vi "Contestant Buzzed.vi"(8 "error in (no error)":errorcluster, 10 "Contestant":i32, 11 "MC Prompt in":refnum<class "MC Prompt.lvclass">) -> (0 "error out":errorcluster, 3 "MC Prompt out":refnum<class "MC Prompt.lvclass">)   [LabVIEW 2021, in "MC Prompt.lvlib" / "MC Prompt.lvclass"]
uses:
  MC Prompt.lvclass
  MC Prompt.lvclass/MC Prompt.ctl
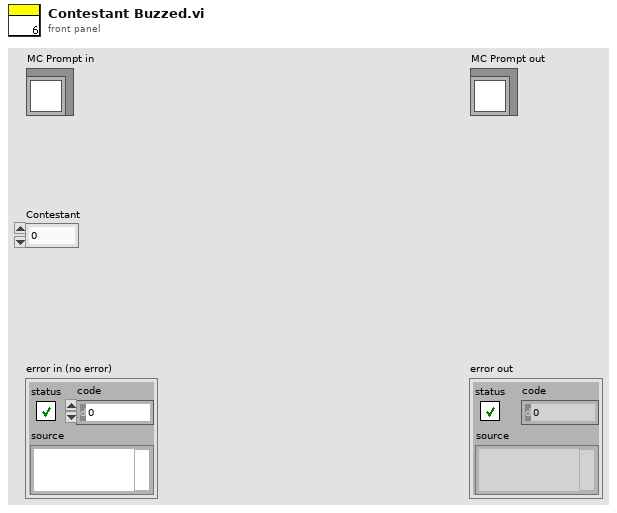
[diagram p1: front panel]
types:
  T1 = enum8{"Enabled", "Disabled", "Disabled and Grayed Out"}
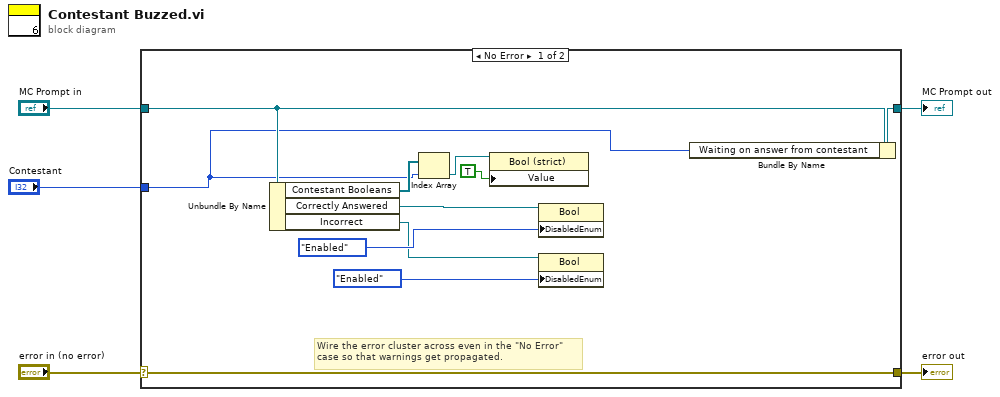
[diagram p0: block diagram]
diagram:
  n1 = case shown="No Error" "error in (no error)" {
    selector: "error in (no error)" -> [w16 w18]
    tunnel: [w16 w18] -> w4
    tunnel: [w7 w17] -> w2
    tunnel: "MC Prompt in" -> [w8 w17]
    tunnel: "Contestant" -> [w6 _]
    frame No Error {
      # "Wire the error cluster across even in the \"No Error\"\ncase so that warnings get propagated."
      n2 = Unbundle By Name(w8) -> ("Contestant Booleans"=w15:refnum<vi>[], "Correctly Answered"=w12:refnum<vi>, "Incorrect"=w9:refnum<vi>)
      n3 = Index Array(array=w15, index=w6) -> (element=w14:refnum<vi>)
      n4 = property class="Bool (strict)"(reference=w14, "Value"=TRUE) -> ()  [unwired: 1 in, 2 out]
      n5 = property class="Bool"(reference=w12, "DisabledEnum"=T1."Enabled" ("Disabled")) -> ()  [unwired: 1 in, 2 out]
      n6 = property class="Bool"(reference=w9, "DisabledEnum"=T1."Enabled" ("Disabled")) -> ()  [unwired: 1 in, 2 out]
      n7 = Bundle By Name(cluster=w8, "Waiting on answer from contestant"=w6) -> (w7:refnum<class "MC Prompt.lvclass">)
    }
    frame Error {
    }
  }
  "error out" <- w4
  "MC Prompt out" <- w2
